vi "DS345_BurstMode.set gate.vi"(0 "i ref in":refnum<vi>, 2 "gate [us]":dbl min=0.0 max=1500.0 step=1.0 format="%.3f", 5 "error in (no error)":errorcluster) -> (14 "i ref out":refnum<vi>, 19 "error out":errorcluster)   [LabVIEW 2014, in "DS345_BurstMode.lvlib"]
doc: "sets the gate value for a DS345. By calling this method, the DS345 can be used as a gate generator that is externally triggered. The delay of the gate pulse delivered is obtained from the \"get delay\" method. The sampling frequency is obtained from the \"get sample freq\" method."
uses:
  DS345_BurstMode.lvlib
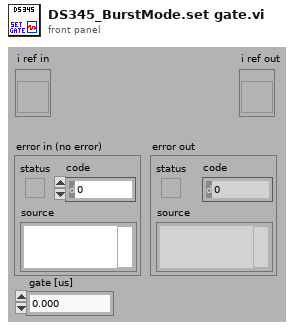
[diagram p1: front panel]
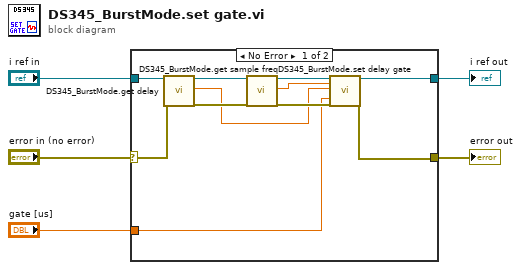
[diagram p0: block diagram]
diagram:
  n1 = case shown="No Error" "error in (no error)" {
    selector: "error in (no error)" -> [w15 w17]
    tunnel: "i ref in" -> [w16 w18]
    tunnel: [w9 w17] -> w4
    tunnel: "gate [us]" -> [w6 _]
    tunnel: [w10 w18] -> w2
    frame No Error {
      n2 = call "DS345_BurstMode.get delay.vi"("i ref in"=w16, "error in (no error)"=w15) -> ("i ref out"=w14:refnum<vi>, "delay [us]"=w7:dbl, "error out"=w13:errorcluster)  [unwired: 15 in]
      n3 = call "DS345_BurstMode.get sample freq.vi"("i ref in"=w14, "error in (no error)"=w13) -> ("i ref out"=w12:refnum<vi>, "sampleFrequency [Hz]"=w8:dbl, "error out"=w11:errorcluster)  [unwired: 15 in]
      n4 = call "DS345_BurstMode.set delay gate.vi"("i ref in"=w12, "sampleFrequency [Hz]"=w8, "delay [us]"=w7, "gate [us]"=w6, "error in (no error)"=w11) -> ("i ref out"=w10:refnum<vi>, "error out"=w9:errorcluster)  [unwired: 13 in]
    }
    frame Error {
    }
  }
  "error out" <- w4
  "i ref out" <- w2
